vi "GetBarStartPosition.vi"(8 "error in (no error)":errorcluster, 11 "EAN-13 in":refnum<class "EAN-13.lvclass">) -> (0 "error out":errorcluster, 2 "Start Position":cluster{"x":i16, "y":i16}={"x"=9, "y"=2}, 3 "EAN-13 out":refnum<class "EAN-13.lvclass">)   [LabVIEW 2013, in "BarCodes.lvlib" / "EAN-13.lvclass"]
doc: "Specifies the top-left corner of the barcode in a given image. This effectively sets the quiet space in either direction around the bar code."
uses:
  EAN-13.lvclass
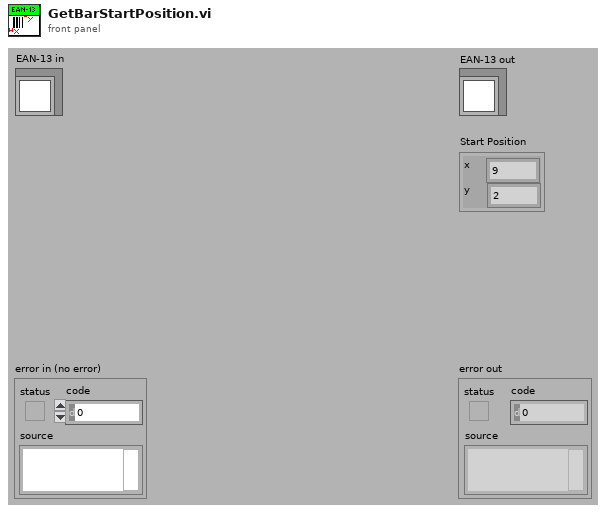
[diagram p1: front panel]
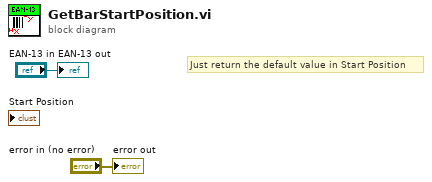
[diagram p0: block diagram]
diagram:
  # "Just return the default value in Start Position"
  "error out" <- "error in (no error)"
  "EAN-13 out" <- "EAN-13 in"
